vi "Device Query.vi"() -> ()   [LabVIEW 2016, in "Generic Device.lvlib" / "Generic Device.lvclass"]
uses:
  Generic Device.lvclass
  <vilib>/Instr/_visa.llb/VISA Find Search Mode.ctl
  SetUp VIs/SetUp VIs.lvlib
panel:
  out "Array":errorcluster[](array[cluster])
  out "Array 2":string[](array[string])
  out "error out 2":errorcluster
  out "Array 3":T1(array[cluster])
  out "Error?":bool[](array[boolean])
  out "Serial Number":string[](array[string])
  out "Device Name":string[](array[string])
  out "Simulated?":bool[](array[boolean])
  out "Product Type":string[](array[string])
  out "Product Category":string[](array[string])
  out "error out":errorcluster
  out "List of Instruments":T1(array[cluster])
  out "# of Instrument Found":i32
  out "find list":string[](array[string])
  in  "error in (no error)":errorcluster
  out "specific error cleared?":bool
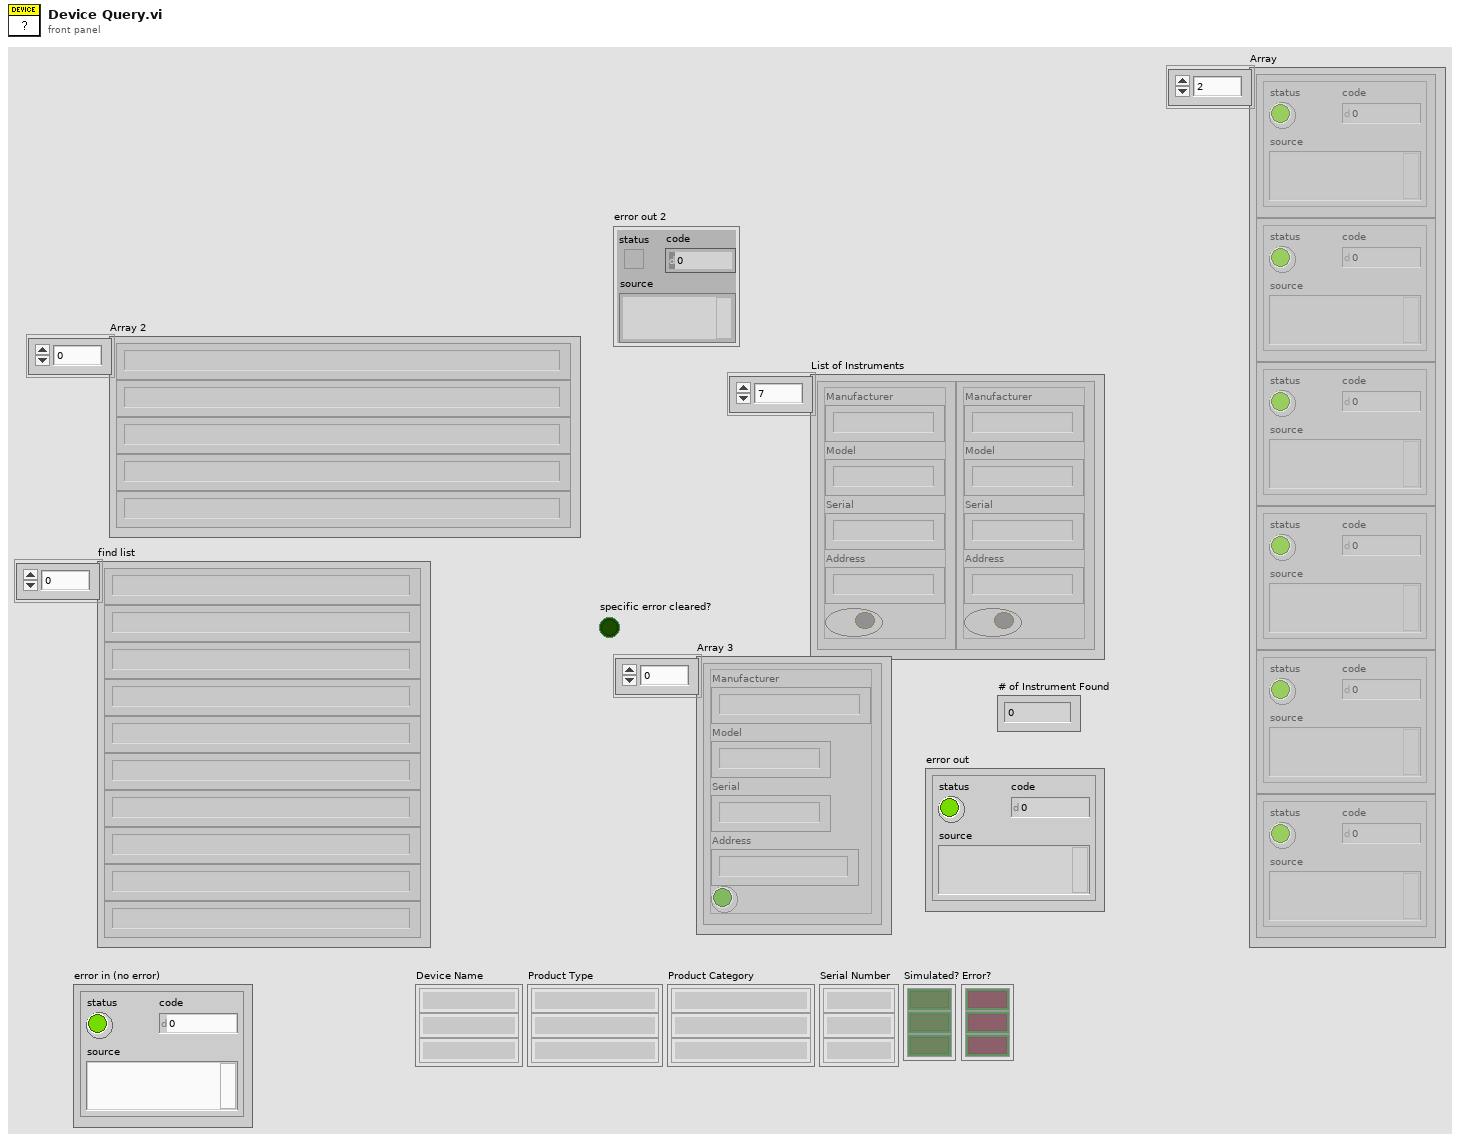
[diagram p1: front panel]
types:
  T1 = cluster{"Manufacturer":string, "Model":string, "Serial":string, "Address":string, "Boolean":bool}[]
  T2 = typedef "VISA Find Search Mode.ctl" = u32
  T3 = cluster{"Manufacturer":string, "Model":string, "Serial":string, "Address":string, bool}[]
  T4 = cluster{"Manufacturer":string, "Model":string, "Serial":string, "Address":string, bool}
  T5 = cluster{"Manufacturer":string, "Model":string, "Serial":string, "Address":string, "Boolean":bool}
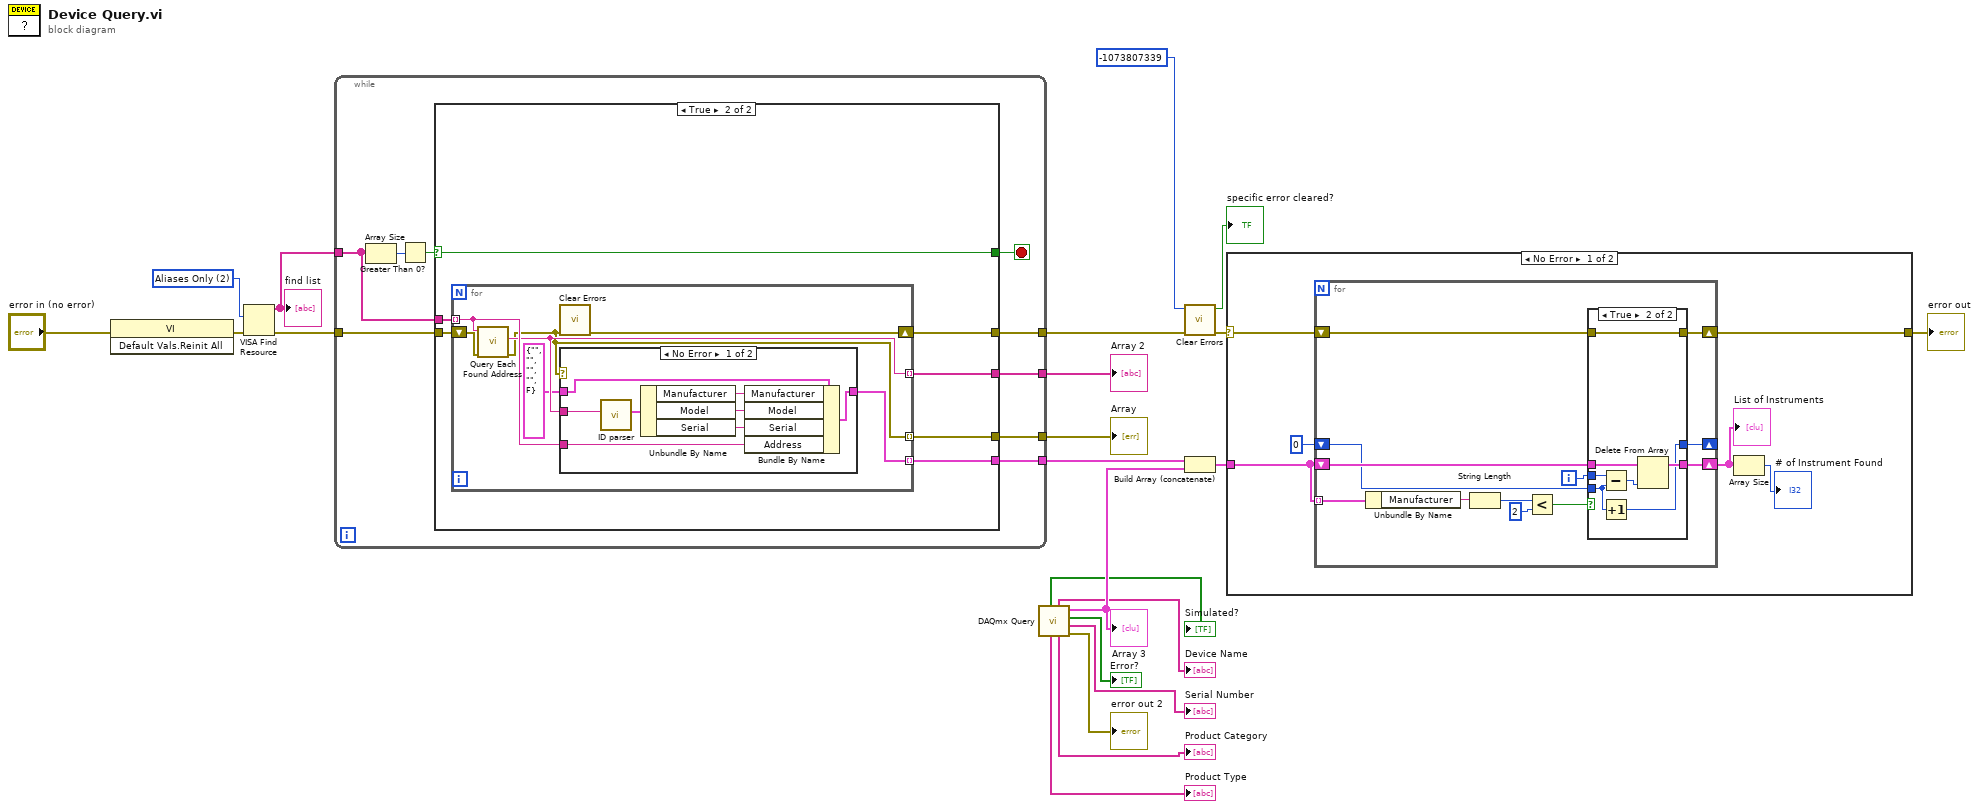
[diagram p0: block diagram]
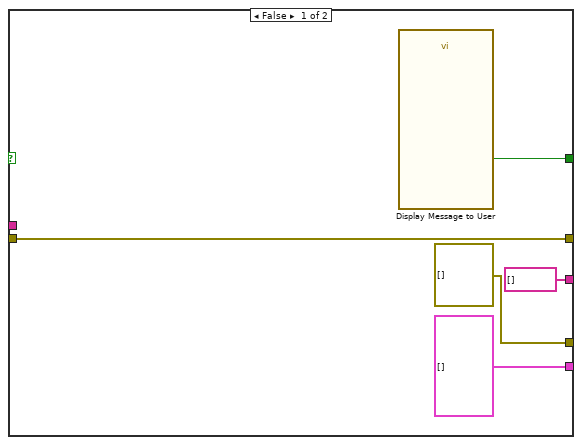
[diagram p4: hidden frame]
diagram:
  w18 = T2 2 items=["Canonical Names Only"=0, "Aliases Only"=2, "Include Matching Aliases"=3, "Include All Aliases"=4] ("Search Mode")
  n1 = invoke class="VI" method="Default Vals.Reinit All"(error in="error in (no error)") -> (error out=w15:errorcluster)  [unwired: 2 in, 2 out]
  n2 = VISA Find Resource(8:w15, 10:w18) -> (0:w16:errorcluster, 3:w19:string[])  [unwired: 1 in, 1 out]
  "find list" <- w19
  n3 = while {
    tunnel: w19 -> [w28]
    tunnel: [w31] -> w21
    tunnel: [w29] -> w11
    tunnel: w16 -> [w30]
    tunnel: [w24] -> w2
    tunnel: [w23] -> w1
    stop <- w25 stop-if-true
    n4 = Array Size(array=w28) -> (size(s)=w27:i32)
    n5 = Greater Than 0?(x=w27) -> (x > 0?=w26:bool)
    n6 = case shown="True" w26 {
      selector: w26 -> [_ w39]
      tunnel: w28 -> [_ w43]
      tunnel: [w35 w42] -> w31
      tunnel: w30 -> [w35 w41]
      tunnel: [T3 [] w40] -> w29
      tunnel: [w36 w39] -> w25
      tunnel: [string[] [] w38] -> w24
      tunnel: [errorcluster[] [] w37] -> w23
      frame False {
        n7 = call "Display Message to User"() -> ("OK"=w36:bool)  [unwired: 10 in, 1 out]
      }
      frame True {
        n8 = for {
          tunnel: w43 -> [w50] mode=indexing
          tunnel: [w49] -> w40 mode=indexing
          shift-right: [w48] -> w42
          shift-left: w41 -> [w45]
          tunnel: [w46] -> w37 mode=indexing
          tunnel: [w47] -> w38 mode=indexing
          n9 = call "Query Each Found Address.vi"("error in (no error) 2"=w45, "VISA resource name out"=w50) -> ("error out (no error)"=w46:errorcluster, "Return String"=w47:string)  [unwired: 8 in]
          n10 = call <vilib>:"Clear Errors.vi"("error in (no error)"=w46) -> ("error out"=w48:errorcluster)  [unwired: 5 in, 1 out]
          n11 = case shown="No Error" w46 {
            tunnel: w50 -> [w58 _]
            tunnel: [w57 w59] -> w49
            tunnel: w47 -> [w56 _]
            tunnel: T4 {"Manufacturer"="", "Model"="", "Serial"="", "Address"="", FALSE} ("Instrument") -> [w55 w59]
            frame No Error {
              n12 = call "ID parser.vi"("Input String"=w56) -> ("output cluster"=w54:T5)  [unwired: 10 in]
              n13 = Unbundle By Name(w54) -> ("Manufacturer"=w53:string, "Model"=w52:string, "Serial"=w51:string)
              n14 = Bundle By Name(cluster=w55, "Manufacturer"=w53, "Model"=w52, "Serial"=w51, "Address"=w58) -> (w57:T4)
            }
            frame Error {
            }
          }
        }
      }
    }
  }
  "Array 2" <- w2
  "Array" <- w1
  n15 = call "DAQmx Query.vi"() -> ("error out"=→"error out 2":errorcluster, "Serial Number"=→"Serial Number":string[], "Error?"=→"Error?":bool[], "Array"=w12:T1, "Product Category"=→"Product Category":string[], "Device Name"=→"Device Name":string[], "Product Type"=→"Product Type":string[], "Simulated?"=→"Simulated?":bool[])  [unwired: 4 in]
  "Array 3" <- w12
  n16 = call <vilib>:"Clear Errors.vi"("error in (no error)"=w21, "specific error code to clear (0: all)"=-1073807339) -> ("error out"=w13:errorcluster, "specific error cleared?"=→"specific error cleared?":bool)  [unwired: 4 in]
  n17 = Build Array (concatenate)(w11, w12) -> (w10:T1)
  n18 = case shown="No Error" w13 {
    selector: w13 -> [w61 w88]
    tunnel: w10 -> [w64 _]
    tunnel: [w60 w88] -> w14
    frame No Error {
      n19 = for {
        tunnel: w64 -> [w77] mode=indexing
        shift-right: [w73] -> w63
        shift-left: w64 -> [w75]
        shift-right: [w67] -> _
        shift-left: 0 -> [w68]
        shift-right: [w66] -> w60
        shift-left: w61 -> [w72]
        i -> [w74]
        n20 = Unbundle By Name(w77) -> ("Manufacturer"=w76:string)
        n21 = String Length(string=w76) -> (length=w69:i32)
        n22 = Less?(x=w69, y=2) -> (x < y?=w71:bool)
        n23 = case shown="True" w71 {
          tunnel: w75 -> [w79 w87]
          tunnel: w74 -> [_ w84]
          tunnel: [w79 w86] -> w73
          tunnel: w72 -> [w80 w85]
          tunnel: [w80 w85] -> w66
          tunnel: w68 -> [w78 w82]
          tunnel: [w78 w81] -> w67
          frame False {
          }
          frame True {
            n24 = Subtract(x=w84, y=w82) -> (x-y=w83:i32)
            n25 = Increment(x=w82) -> (x+1=w81:i32)
            n26 = Delete From Array(array=w87, index=w83) -> (array with subset deleted=w86:T1)  [unwired: 1 in, 1 out]
          }
        }
      }
      "List of Instruments" <- w63
      n27 = Array Size(array=w63) -> (size(s)=→"# of Instrument Found":i32)
    }
    frame Error {
    }
  }
  "error out" <- w14
